vi "Method.vi"(4 "Input B":refnum<class "Abs_Numeric.lvclass">, 5 "Input A":refnum<class "Abs_U16 Integer.lvclass">) -> (1 "Result":T1)   [LabVIEW 2021, in "Subtract_U16.lvclass"]
uses:
  Subtract_U16.lvclass
  Abs_Types/U16 Integer/Abs_U16 Integer.lvclass
  Abs Type.ctl
  Abs_Types/Numeric/Abs_Numeric.lvclass
  C:/TSA/LV_Abstract/Source/Functions/Support/Function/Two Terminal/U16/AbsFunc_Two Term_U16.lvclass
  C:/Program Files (x86)/National Instruments/LabVIEW 2021/vi.lib/TSA/Abstract Data Classes/Abs_Types/U16 Integer/Abs_U16 Integer.lvclass
  Support/Function/Two Terminal/U16/AbsFunc_Two Term_U16.lvclass/AbsFunc_Two Term_U16.ctl
  Support/Function/Two Terminal/U16/Properties/Write Numeric A.vi
  Support/Function/Two Terminal/U16/Properties/Write Numeric B.vi
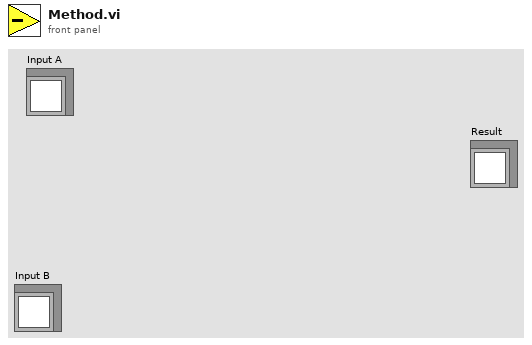
[diagram p1: front panel]
types:
  T1 = typedef "Subtract_U16.lvclass/Abs Type.ctl" = refnum<class "Abs_U16 Integer.lvclass">
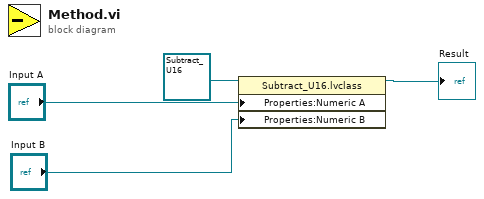
[diagram p0: block diagram]
diagram:
  n1 = property class="Subtract_U16.lvclass"(reference=refnum<class "Subtract_U16.lvclass"> refnum ("Subtract_DBL.lvclass"), "Properties:Numeric A"="Input A", "Properties:Numeric B"="Input B") -> (reference out=→"Result":refnum<class "Subtract_U16.lvclass">)  [unwired: 1 in, 1 out]
